vi "Reason Master.vi"(8 "error in (no error)":errorcluster) -> (0 "error out":errorcluster)   [LabVIEW 2017]
uses:
  <vilib>/addons/database/Connection.llb/DB Tools Open Connec (Path).vi
  <vilib>/addons/database/NI_Database_API.lvlib
panel:
  in  "Cancel Button - Archive":bool
  out "data":string[][](array[string])
  in  "Select Stakeholder":string(combo)
  in  "Select Station 2":string(combo)
  in  "Delete Reason":bool
  in  "Select Stakeholder 2":string(combo)
  in  "Select Station":string(combo)
  in  "Get Reason":bool
  in  "Add Reason":string
  out "Table":string[][](table)
  in  "Add Reason":bool
  # "Add Reason"
  # "View Reasons"
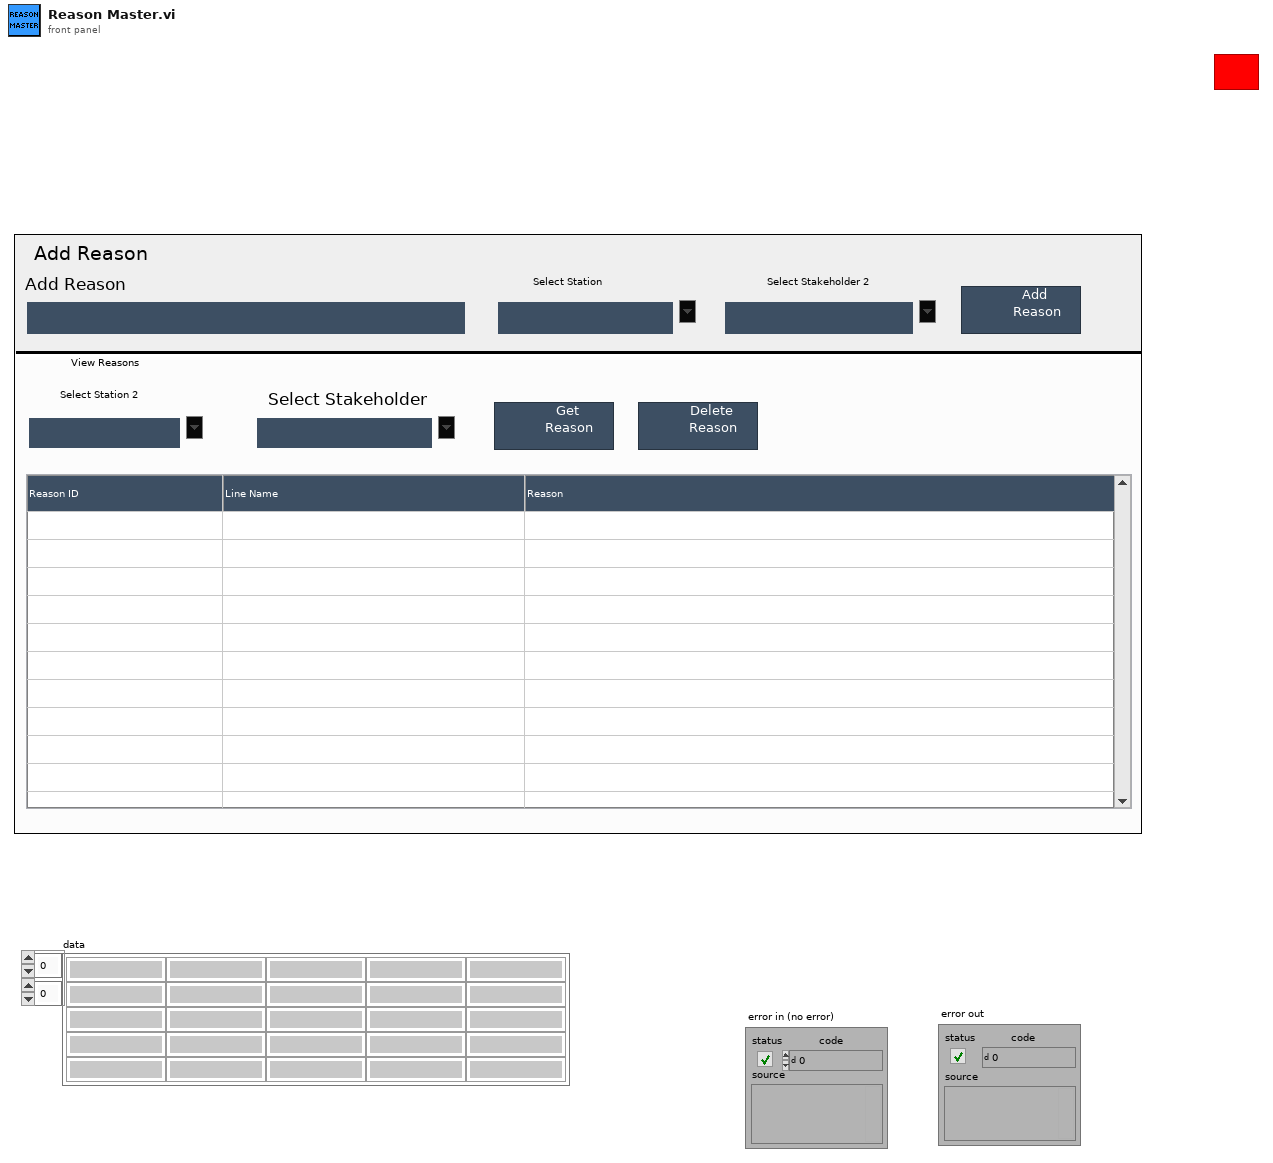
[diagram p1: front panel]
types:
  T1 = typedef "NI_Database_API.lvlib/Conn ObjectReference.ctl" = refnum<k1>
  T2 = enum32{"invalid app kind", "Development System", "Run Time System", "Student Edition", "Embedded LabVIEW", "Evaluation", "Custom"}
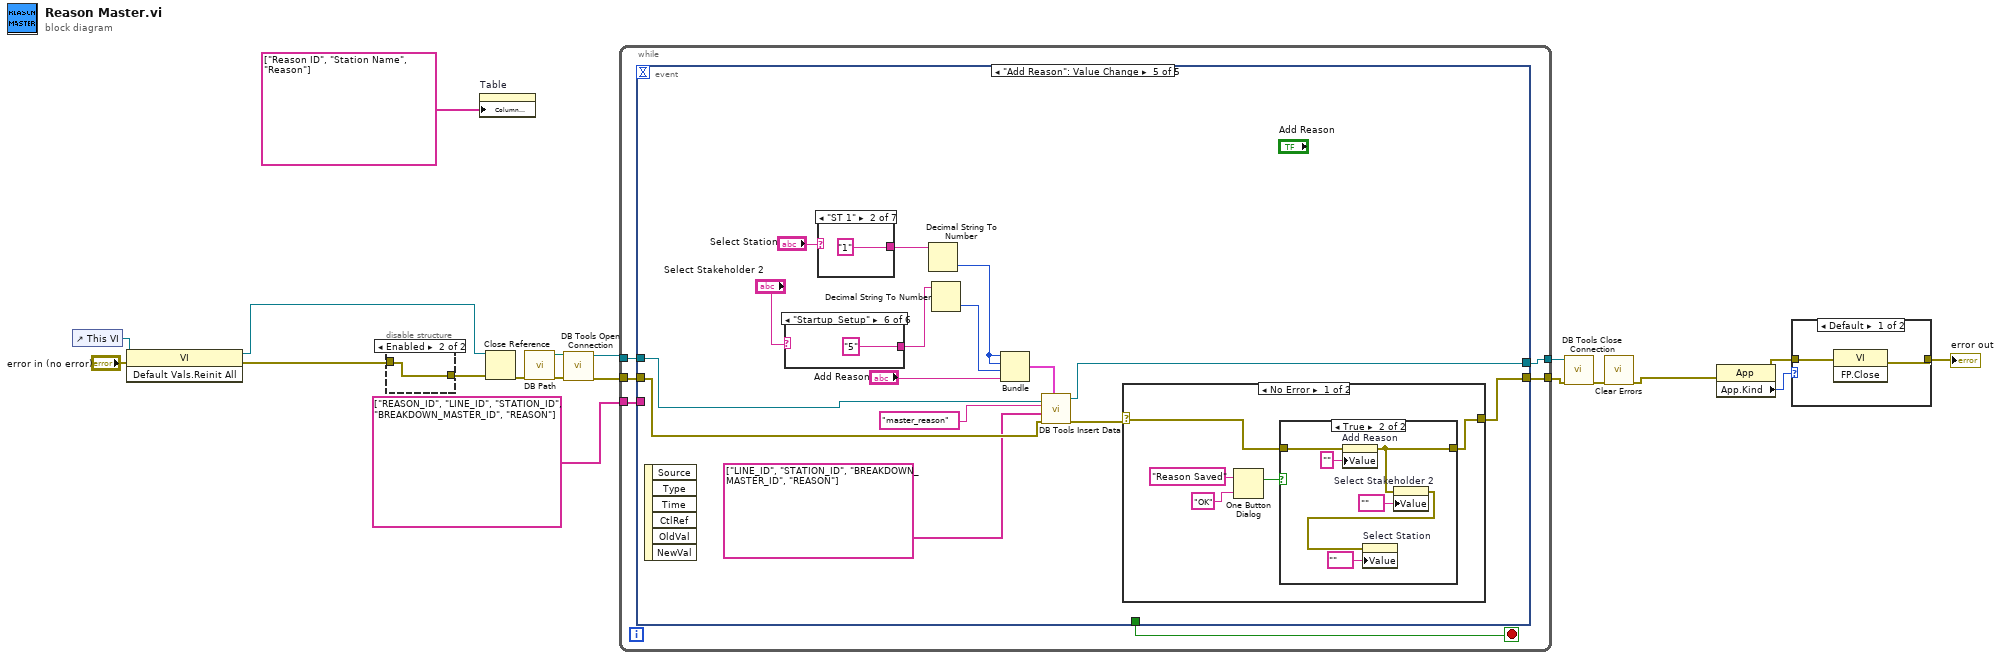
[diagram p0: block diagram]
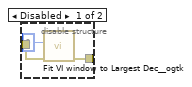
[diagram p2: hidden frame]
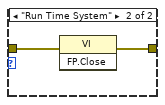
[diagram p3: hidden frame]
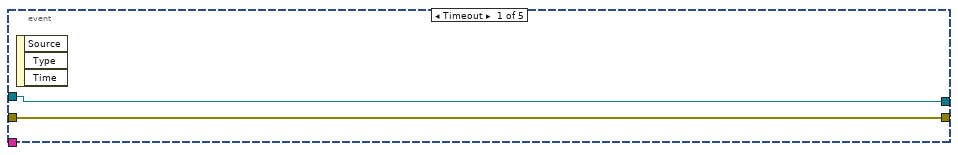
[diagram p4: hidden frame]
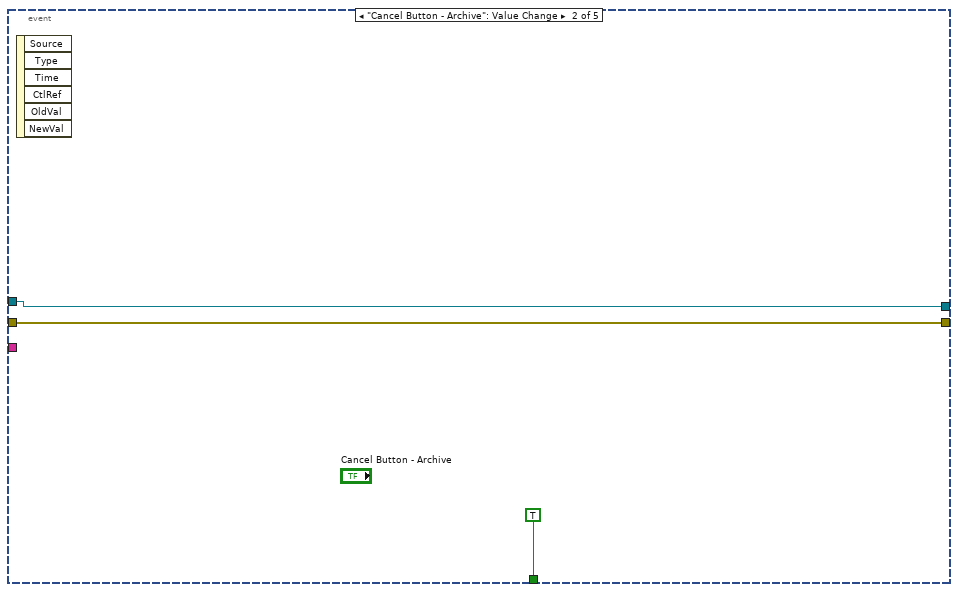
[diagram p5: hidden frame]
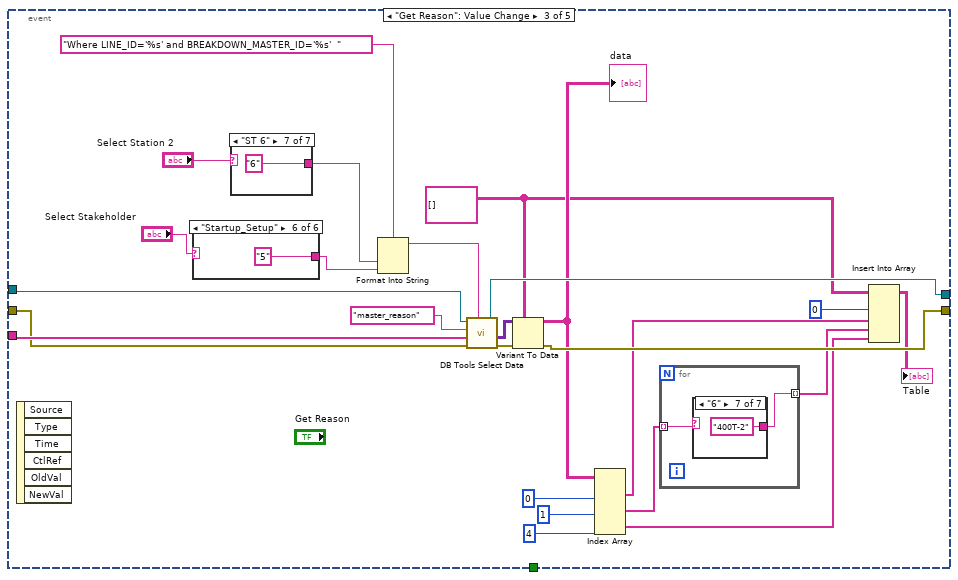
[diagram p6: hidden frame]
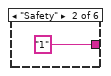
[diagram p8: hidden frame]
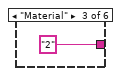
[diagram p9: hidden frame]
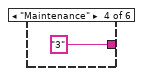
[diagram p10: hidden frame]
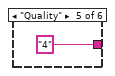
[diagram p11: hidden frame]
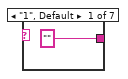
[diagram p12: hidden frame]
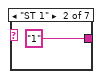
[diagram p13: hidden frame]
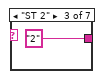
[diagram p14: hidden frame]
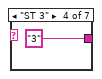
[diagram p15: hidden frame]
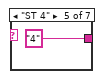
[diagram p16: hidden frame]
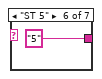
[diagram p17: hidden frame]
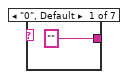
[diagram p18: hidden frame]
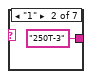
[diagram p19: hidden frame]
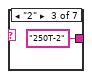
[diagram p20: hidden frame]
diagram:
  n1 = control-ref of="This VI"() -> (w19:refnum<vi>)
  n2 = invoke class="VI" method="Default Vals.Reinit All"(reference=w19, error in="error in (no error)") -> (reference out=w17:refnum<vi>, error out=w5:errorcluster)  [unwired: 1 in, 1 out]
  n3 = disable-structure shown="Enabled" {
    disable-tunnel: w5 -> [w22 w23]
    disable-tunnel: [w21 w23] -> w4
    frame Disabled {
      n4 = call <userlib>:"Fit VI window to Largest Dec__ogtk.vi"("error in (no error)"=w22, "border spacing (2 px)"=0) -> ("error out"=w21:errorcluster)  [unwired: 4 in, 1 out]
    }
    frame Enabled {
    }
  }
  n5 = property on="Table" class="Tbl (strict)"("Column Headers[]"=string[] ["Reason ID", "Station Name", "Reason"] ("Column Header Strings[]")) -> ()  [unwired: 2 in, 2 out]
  n6 = Close Reference(reference=w17, error in (no error)=w4) -> (error out=w13:errorcluster)
  n7 = call "DB Path.vi"("error in"=w13) -> ("error out"=w15:errorcluster, "DB Path"=w14:path)  [unwired: 9 in]
  n8 = call-poly <vilib>:"DB Tools Open Connection.vi"("error in (no error)"=w15, "connection information"=w14) -> ("error out"=w12:errorcluster, "connection reference"=w10:T1)  [unwired: 6 in]
  n9 = while {
    tunnel: w12 -> [w29]
    tunnel: [w27] -> w7
    tunnel: string[] ["REASON_ID", "LINE_ID", "STATION_ID", "BREAKDOWN_MASTER_ID", "REASON"] ("Table") -> [w26]
    tunnel: w10 -> [w25]
    tunnel: [w24] -> w6
    stop <- w28 stop-if-true
    n10 = event shown="[4] \"Add Reason\": Value Change" {
      selector: _ -> [_ _ _ _ _]
      dyn-events: _ -> [_ _ _ _ _]
      timeout: _ -> [_ _ _ _ _]
      tunnel: w29 -> [w30 w32 w51 w106 w140]
      tunnel: [_ TRUE _ _ _] -> w28
      tunnel: [w30 w32 w52 w85 w132] -> w27
      tunnel: w26 -> [_ _ w59 w87 _]
      tunnel: w25 -> [w31 w33 w57 w107 w141]
      tunnel: [w31 w33 w50 w86 w138] -> w24
      event Timeout {
        n11 = event-data() -> ()  [unwired: 1 in, 3 out]
      }
      event "Cancel Button - Archive": Value Change {
        n12 = event-data() -> ()  [unwired: 1 in, 6 out]
      }
      event "Get Reason": Value Change {
        w46 = string[][] []
        n13 = event-data() -> ()  [unwired: 1 in, 6 out]
        n14 = case shown="\"Startup_Setup\"" "Select Stakeholder" {
          tunnel: [_ "1" "2" "3" "4" "5"] -> w35
          frame "False", Default {
          }
          frame "Safety" {
          }
          frame "Material" {
          }
          frame "Maintenance" {
          }
          frame "Quality" {
          }
          frame "Startup_Setup" {
          }
        }
        n15 = case shown="\"ST 6\"" "Select Station 2" {
          tunnel: ["" "1" "2" "3" "4" "5" "6"] -> w37
          frame "1", Default {
          }
          frame "ST 1" {
          }
          frame "ST 2" {
          }
          frame "ST 3" {
          }
          frame "ST 4" {
          }
          frame "ST 5" {
          }
          frame "ST 6" {
          }
        }
        n16 = Format Into String(format string="Where LINE_ID='%s' and BREAKDOWN_MASTER_ID='%s'  " ("condition"), w37, w35) -> (resulting string=w56:string)  [unwired: 2 in, 1 out]
        n17 = call <vilib>:"DB Tools Select Data.vi"("condition"=w56, "error in (no error)"=w51, "columns"=w59, "table"="master_reason", "connection reference"=w57) -> ("error out"=w53:errorcluster, "data"=w54:variant[][], "connection reference out"=w50:T1)  [unwired: 1 in]
        n18 = Variant To Data(error in=w53, type=w46, Variant=w54) -> (data=w47:string[][], error out=w52:errorcluster)
        "data" <- w47
        n19 = Index Array(array=w47, index (col) #1=0 ("disabled index (col)"), index (col) #2=1 ("disabled index (col)"), index (col) #3=4 ("index (col)")) -> (element #1=w39:string[], element #2=w42:string[], element #3=w44:string[])  [unwired: 3 in]
        n20 = for {
          tunnel: w42 -> [w73] mode=indexing
          tunnel: [w72] -> w41 mode=indexing
          n21 = case shown="\"6\"" w73 {
            tunnel: ["" "250T-3" "250T-2" "250T-1" "400T-1" "150T-1" "400T-2"] -> w72
            frame "0", Default {
            }
            frame "1" {
            }
            frame "2" {
            }
            frame "3" {
            }
            frame "4" {
            }
            frame "5" {
            }
            frame "6" {
            }
          }
        }
        n22 = Insert Into Array(array=w46, index (col)=0 ("disabled index (col)"), new element #1=w39, new element #2=w41, new element #3=w44) -> (→"Table":string[][])  [unwired: 1 in]
      }
      event "Delete Reason": Value Change {
        w98 = string[][] []
        n23 = event-data() -> ()  [unwired: 1 in, 6 out]
        n24 = local read "Select Station 2"() -> (w82:string)
        n25 = local read "Select Stakeholder"() -> (w83:string)
        n26 = call "DELETE REASON.vi"("error in (no error)"=w106, "connection reference"=w107) -> ("error out"=w89:errorcluster, "connection reference out"=w90:T1)  [unwired: 8 in]
        n27 = case shown="\"ST 1\"" w82 {
          tunnel: ["" "1" "2" "3" "4" "5" "6"] -> w81
          frame "1", Default {
          }
          frame "ST 1" {
          }
          frame "ST 2" {
          }
          frame "ST 3" {
          }
          frame "ST 4" {
          }
          frame "ST 5" {
          }
          frame "ST 6" {
          }
        }
        n28 = case shown="\"Startup_Setup\"" w83 {
          tunnel: [_ "1" "2" "3" "4" "5"] -> w93
          frame "False", Default {
          }
          frame "Safety" {
          }
          frame "Material" {
          }
          frame "Maintenance" {
          }
          frame "Quality" {
          }
          frame "Startup_Setup" {
          }
        }
        n29 = Format Into String(format string="Where LINE_ID='%s' and BREAKDOWN_MASTER_ID='%s'  " ("condition"), w81, w93) -> (resulting string=w105:string)  [unwired: 2 in, 1 out]
        n30 = call <vilib>:"DB Tools Select Data.vi"("condition"=w105, "error in (no error)"=w89, "columns"=w87, "table"="master_reason", "connection reference"=w90) -> ("error out"=w102:errorcluster, "data"=w103:variant[][], "connection reference out"=w86:T1)  [unwired: 1 in]
        n31 = Variant To Data(error in=w102, type=w98, Variant=w103) -> (data=w99:string[][], error out=w85:errorcluster)
        n32 = Index Array(array=w99, index (col) #1=0 ("disabled index (col)"), index (col) #2=1 ("disabled index (col)"), index (col) #3=4 ("index (col)")) -> (element #1=w91:string[], element #2=w95:string[], element #3=w96:string[])  [unwired: 3 in]
        n33 = for {
          tunnel: w95 -> [w116] mode=indexing
          tunnel: [w115] -> w94 mode=indexing
          n34 = case shown="\"0\", Default" w116 {
            tunnel: ["" "250T-3" "250T-2" "250T-1" "400T-1" "150T-1" "400T-2"] -> w115
            frame "0", Default {
            }
            frame "1" {
            }
            frame "2" {
            }
            frame "3" {
            }
            frame "4" {
            }
            frame "5" {
            }
            frame "6" {
            }
          }
        }
        n35 = Insert Into Array(array=w98, index (col)=0 ("disabled index (col)"), new element #1=w91, new element #2=w94, new element #3=w96) -> (w84:string[][])  [unwired: 1 in]
        n36 = property on="Table" class="Tbl (strict)"("Value"=w84) -> ()  [unwired: 2 in, 2 out]
      }
      event "Add Reason": Value Change {
        n37 = event-data() -> ()  [unwired: 1 in, 6 out]
        n38 = case shown="\"Startup_Setup\"" "Select Stakeholder 2" {
          tunnel: [_ "1" "2" "3" "4" "5"] -> w130
          frame "False", Default {
          }
          frame "Safety" {
          }
          frame "Material" {
          }
          frame "Maintenance" {
          }
          frame "Quality" {
          }
          frame "Startup_Setup" {
          }
        }
        n39 = case shown="\"ST 1\"" "Select Station" {
          tunnel: ["" "1" "2" "3" "4" "5" "6"] -> w135
          frame "1", Default {
          }
          frame "ST 1" {
          }
          frame "ST 2" {
          }
          frame "ST 3" {
          }
          frame "ST 4" {
          }
          frame "ST 5" {
          }
          frame "ST 6" {
          }
        }
        n40 = Decimal String To Number(string=w135) -> (number=w131:i32)  [unwired: 2 in, 1 out]
        n41 = Decimal String To Number(string=w130) -> (number=w134:i32)  [unwired: 2 in, 1 out]
        n42 = Bundle(w131, w131, w134, "Add Reason"="Add Reason") -> (w142:cluster{i32, i32, i32, "Add Reason":string})  [unwired: 1 in]
        n43 = call <vilib>:"DB Tools Insert Data.vi"("data"=w142, "error in (no error)"=w140, "columns"=string[] ["LINE_ID", "STATION_ID", "BREAKDOWN_MASTER_ID", "REASON"] ("Table"), "table"="master_reason", "connection reference"=w141) -> ("error out"=w133:errorcluster, "connection reference out"=w138:T1)  [unwired: 5 in]
        n44 = case shown="No Error" w133 {
          selector: w133 -> [w150 w161]
          tunnel: [w149 w161] -> w132
          frame No Error {
            n45 = One Button Dialog(message="Reason Saved", button name ("OK")="OK") -> (true=w151:bool)
            n46 = case shown="True" w151 {
              tunnel: w150 -> [w154 w159]
              tunnel: [w154 w158] -> w149
              frame False {
              }
              frame True {
                n47 = property on="Add Reason" class="Str"(error in=w159, "Value"="" ("Add Reason")) -> (error out=w158:errorcluster)  [unwired: 1 in, 1 out]
                n48 = property on="Select Stakeholder 2" class="CmbBox"(error in=w158, "Value"="" ("Select Stakeholder 2")) -> (error out=w156:errorcluster)  [unwired: 1 in, 1 out]
                n49 = property on="Select Station" class="CmbBox"(error in=w156, "Value"="" ("Select Station")) -> ()  [unwired: 1 in, 2 out]
              }
            }
          }
          frame Error {
            n50 = One Button Dialog(message="Reason Not Saved", button name ("OK")="OK") -> ()  [unwired: 1 out]
          }
        }
      }
    }
  }
  n51 = call <vilib>:"DB Tools Close Connection.vi"("error in (no error)"=w7, "connection reference"=w6) -> ("error out"=w9:errorcluster)  [unwired: 5 in]
  n52 = call <vilib>:"Clear Errors.vi"("error in (no error)"=w9) -> ("error out"=w8:errorcluster)  [unwired: 5 in, 1 out]
  n53 = property class="App"(error in=w8) -> (error out=w2:errorcluster, "App.Kind"=w3:T2)  [unwired: 1 in, 1 out]
  n54 = case shown="Default" w3 {
    tunnel: w2 -> [w172 w174]
    tunnel: [w171 w173] -> w16
    frame Default {
      n55 = invoke class="VI" method="FP.Close"(error in=w172) -> (error out=w171:errorcluster)  [unwired: 2 in, 2 out]
    }
    frame "Run Time System" {
      n56 = invoke class="VI" method="FP.Close"(error in=w174) -> (error out=w173:errorcluster)  [unwired: 2 in, 2 out]
    }
  }
  "error out" <- w16
